vi "merFISH_piezo_autofocus_security.vi"(3 "error in":errorcluster, 4 "queue piezo":refnum<queue>, 5 "queue ASI stage":refnum<queue>) -> (0 "error out":errorcluster)   [LabVIEW 2015]
uses:
  CONTROLS/Q_MCL_piezo_element.ctl
  CONTROLS/Q_ASI_stage_element.ctl
  GLOBAL/Global_MCL_piezo.vi
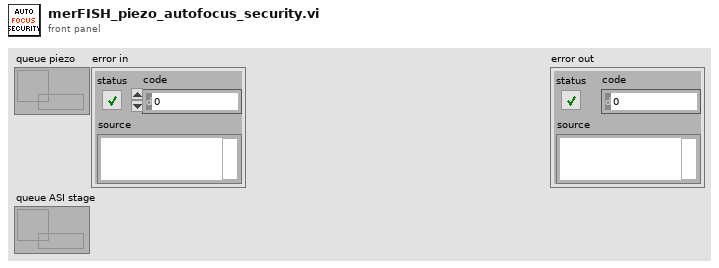
[diagram p1: front panel]
types:
  T1 = typedef "Q_MCL_piezo_element.ctl" = cluster{"variant":variant, "Instruction":enum16{"Piezo_idle", "Piezo_initialize", "Piezo_error", "Piezo_security_stop", "Piezo_read_z", "Piezo_move_z", "Piezo_keyboard_move", "Piezo_close_autofocus_calibration_ramp", "Piezo_change_init_state", "Piezo_init_autofocus", "Piezo_init_autofocus_merFISH_TL", "Piezo_autofocus", "Piezo_autofocus_merFISH_TL", "Piezo_stop_autofocus", "Piezo_stop_autofocus_merFISH_TL", "Piezo_autofocus_lost", "Piezo_resume_autofocus_merFISH_TL", "Piezo_check_z_position_merFISH_TL", "Piezo_init_ramp", "Piezo_move_z_ramp", "Piezo_close_ramp", "Piezo_close_merFISH", "Piezo_init_TL", "Piezo_close_ramp_TL", "Piezo_close_TL", "Piezo_stop"}}
  T2 = typedef "Q_ASI_stage_element.ctl" = cluster{"variant":variant, "Instruction":enum16{"ASI_idle", "ASI_initialize", "ASI_error", "ASI_security_stop", "ASI_read_XYZ", "ASI_up", "ASI_down", "ASI_left", "ASI_right", "ASI_save_XY", "ASI_move_to_XY", "ASI_brightfield", "ASI_init_scan", "ASI_init_merFISH", "ASI_move_to_XY_merFISH", "ASI_move_to_Z_merFISH", "ASI_init_autofocus_search_merFISH", "ASI_close_autofocus_search_merFISH", "ASI_adjust_piezo_autofocus_merFISH", "ASI_set_piezo_autofocus_to_reference_position_merFISH_TL", "ASI_close_merFISH", "ASI_init_TL", "ASI_move_mosaic_TL", "ASI_brightfield_TL", "ASI_close_TL", "ASI_stop"}}
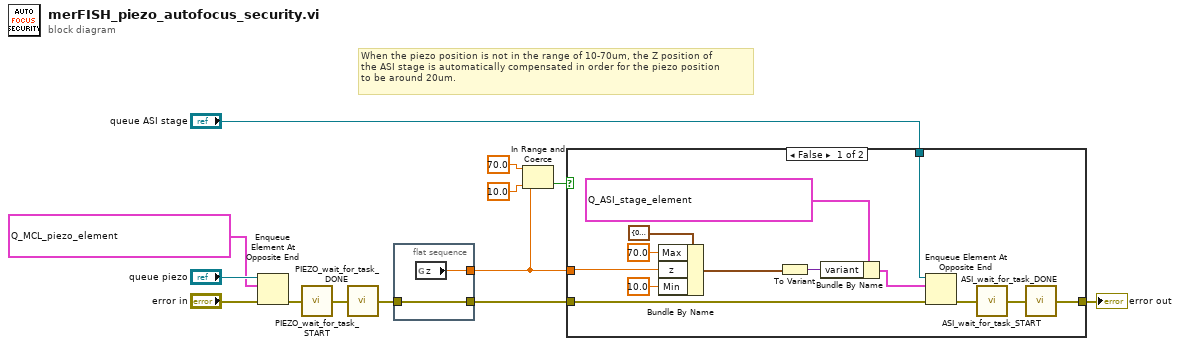
[diagram p0: block diagram]
diagram:
  # "When the piezo position is not in the range of 10-70um, the Z position of\nthe ASI stage is automatically compensated in order for the piezo position \nto be around 20um."
  n1 = Enqueue Element At Opposite End(queue="queue piezo", element=T1 {"variant"=variant, "Instruction"=enum."Piezo_check_z_position_merFISH_TL"}, error in (no error)="error in") -> (error out=w10:errorcluster)  [unwired: 1 in, 2 out]
  n2 = call "PIEZO_wait_for_task_START.vi"("error in"=w10) -> ("error out"=w9:errorcluster)
  n3 = call "PIEZO_wait_for_task_DONE.vi"("error in"=w9) -> ("error out"=w8:errorcluster)
  n4 = flat-sequence {
    tunnel: w8 -> [w15]
    tunnel: [w15] -> w4
    tunnel: [w14] -> w1
    frame #0 {
      n5 = global read "Global_MCL_piezo.vi" "z"() -> (w14:dbl)
    }
  }
  n6 = In Range and Coerce(upper limit=70.0, x=w1, lower limit=10.0 ("upper limit")) -> (In Range?=w5:bool)  [unwired: 1 out]
  n7 = case shown="False" w5 {
    tunnel: w4 -> [w28 w29]
    tunnel: "queue ASI stage" -> [w27 _]
    tunnel: [w24 w29] -> w2
    tunnel: w1 -> [w19 _]
    frame False {
      n8 = Bundle By Name(cluster=cluster{"Min":dbl, "Max":dbl, "z":dbl} {"Min"=0.0, "Max"=0.0, "z"=0.0} ("Limits"), "Max"=70.0, "z"=w19, "Min"=10.0) -> (w16:cluster{"Min":dbl, "Max":dbl, "z":dbl})
      n9 = To Variant(anything=w16) -> (Variant=w22:variant)
      n10 = Bundle By Name(cluster=T2 {"variant"=variant, "Instruction"=enum."ASI_adjust_piezo_autofocus_merFISH"} ("element"), "variant"=w22) -> (w21:T2)
      n11 = Enqueue Element At Opposite End(queue=w27, element=w21, error in (no error)=w28) -> (error out=w26:errorcluster)  [unwired: 1 in, 2 out]
      n12 = call "ASI_wait_for_task_START.vi"("error in"=w26) -> ("error out"=w25:errorcluster)
      n13 = call "ASI_wait_for_task_DONE.vi"("error in"=w25) -> ("error out"=w24:errorcluster)
    }
    frame True {
    }
  }
  "error out" <- w2
